vi "Test.vi"() -> ()   [LabVIEW 2012]
uses:
  Opening Purpose.ctl
panel:
  out "Number of Pages":i32
  out "error out":errorcluster
  in  "Original File Path":path
  in  "Opening Purpose":T1
  in  "TIFF File Path":path
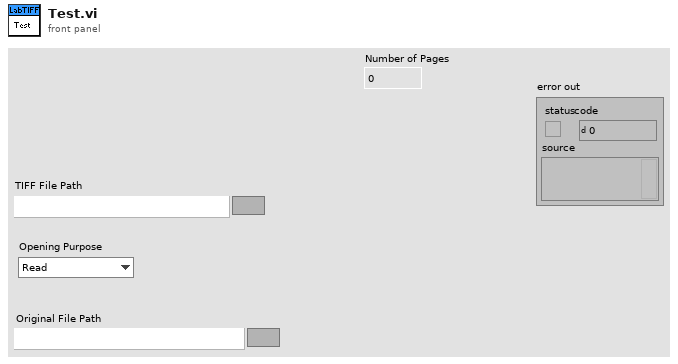
[diagram p1: front panel]
types:
  T1 = typedef "Opening Purpose.ctl" = enum16{"Read", "Write"}
  T2 = typedef "Image Type" = u32
  T3 = typedef "IMAQ Image.ctl" = refnum<image>
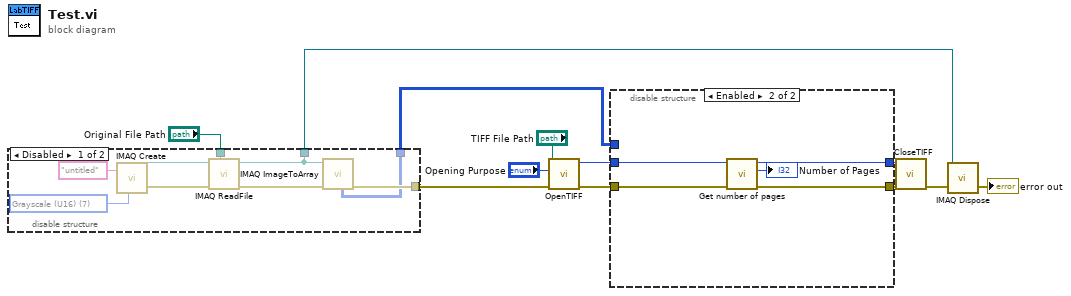
[diagram p0: block diagram]
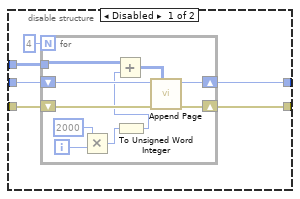
[diagram p2: hidden frame]
diagram:
  n1 = disable-structure shown="Disabled" {
    disable-tunnel: "Original File Path" -> [w17 _]
    disable-tunnel: [w15 _] -> w9
    disable-tunnel: [w14 _] -> w3
    disable-tunnel: [w13 _] -> w1
    frame Disabled {
      w18 = T2 7 items=["Grayscale (U8)", "Grayscale (I16)", "Grayscale (SGL)", "Complex (CSG)", "RGB (U32)", "HSL (U32)", "RGB (U64)", "Grayscale (U16)"] ("Image Type")
      n2 = call "IMAQ Create"("Image Name"="untitled", "Image Type"=w18) -> ("New Image"=w20:T3, "error out"=w19:errorcluster)  [unwired: 3 in]
      n3 = call "IMAQ ReadFile"("File Path"=w17, "error in (no error)"=w19, "Image"=w20) -> ("error out"=w16:errorcluster, "Image Out"=w14:T3)  [unwired: 4 in, 3 out]
      n4 = call "IMAQ ImageToArray"("error in (no error)"=w16, "Image"=w14) -> ("Image Pixels (U16)"=w13:u16[][], "error out"=w15:errorcluster)  [unwired: 2 in, 3 out]
    }
    frame Enabled {
    }
  }
  n5 = call "OpenTIFF.vi"("error in (no error)"=w9, "Opening Purpose"="Opening Purpose", "File Path"="TIFF File Path") -> ("error out"=w8:errorcluster, "TIFF File Ref"=w7:i32)  [unwired: 7 in]
  n6 = disable-structure shown="Enabled" {
    disable-tunnel: w8 -> [w27 w40]
    disable-tunnel: w7 -> [w26 w42]
    disable-tunnel: [w25 w41] -> w6
    disable-tunnel: [w24 w39] -> w5
    disable-tunnel: w1 -> [w23 _]
    frame Disabled {
      n7 = for {
        N: 4 -> [_]
        tunnel: w23 -> [w31]
        shift-right: [w35] -> w24
        shift-left: w27 -> [w37]
        shift-right: [w36] -> w25
        shift-left: w26 -> [w32]
        i -> [w34]
        n8 = Multiply(x=2000, y=w34) -> (x*y=w30:i32)
        n9 = To Unsigned Word Integer(number=w30) -> (unsigned 16bit integer=w29:u16)
        n10 = Add(x=w31, y=w29) -> (x+y=w28:u16[][])
        n11 = call "Append Page.vi"("U16 Image"=w28, "error in (no error)"=w37, "TIFF File Ref"=w32) -> ("error out"=w35:errorcluster, "TIFF File Ref out"=w36:i32)  [unwired: 7 in]
      }
    }
    frame Enabled {
      n12 = call "Get number of pages.vi"("error in (no error)"=w40, "TIFF File ref"=w42) -> ("error out"=w39:errorcluster, "Number of Pages"=→"Number of Pages":i32, "TIFF File ref out"=w41:i32)  [unwired: 7 in]
    }
  }
  n13 = call "CloseTIFF.vi"("error in (no error)"=w5, "TIFF File Ref"=w6) -> ("error out"=w4:errorcluster)  [unwired: 9 in]
  n14 = call "IMAQ Dispose"("Image"=w3, "error in (no error)"=w4) -> ("error out"=→"error out":errorcluster)  [unwired: 4 in]
